vi "WriteRegen.vi"(3 "error in (no error)":errorcluster, 5 "task in":refnum<k24>) -> (0 "error out":errorcluster, 1 "Regenerate":bool, 2 "task out":refnum<k24>)   [LabVIEW 2010]
uses:
  C:/Program Files/National Instruments/LabVIEW 2010/vi.lib/ULx/ULx_LV.dll
  Program Files/National Instruments/LabVIEW 2010/vi.lib/ULx/ULx_LV.dll
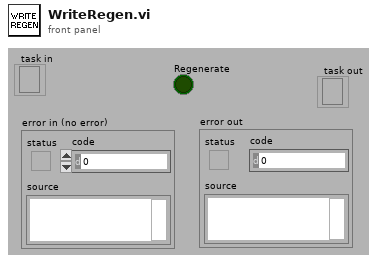
[diagram p1: front panel]
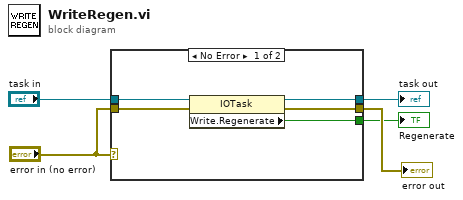
[diagram p0: block diagram]
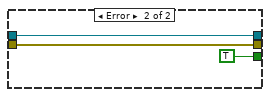
[diagram p2: hidden frame]
diagram:
  n1 = case shown="No Error" "error in (no error)" {
    tunnel: "task in" -> [w8 w13]
    tunnel: "error in (no error)" -> [w9 w12]
    tunnel: [w6 w13] -> w4
    tunnel: [w7 w12] -> w3
    tunnel: [w10 TRUE ("Read.AutoStart")] -> w1
    frame No Error {
      n2 = property class="IOTask"(reference=w8, error in=w9) -> (reference out=w6:refnum<k24>, error out=w7:errorcluster, "Write.Regenerate"=w10:bool)
    }
    frame Error {
    }
  }
  "task out" <- w4
  "error out" <- w3
  "Regenerate" <- w1
